vi "Client.vi"() -> ()   [LabVIEW 2025]
panel:
  in  "Stop":bool
  out "Waveform Chart":dbl(graph)
  out "Alarm Message":string
  out "Alarm LED":bool
  out "Max Temp":dbl
  out "Min Temp":dbl
  out "Moving Avg":dbl
  out "Current Temp":dbl
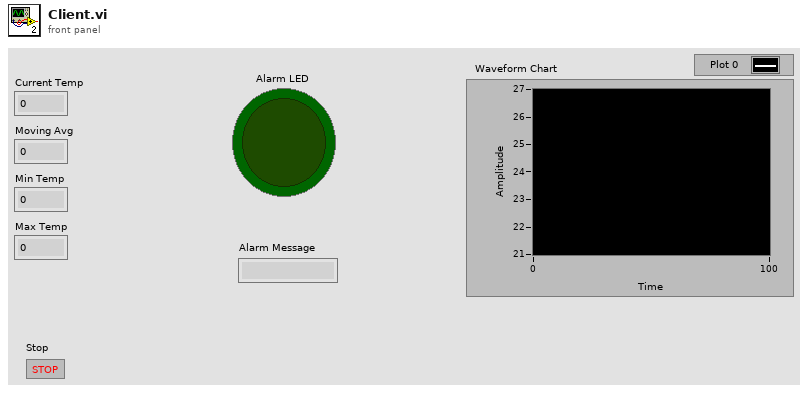
[diagram p1: front panel]
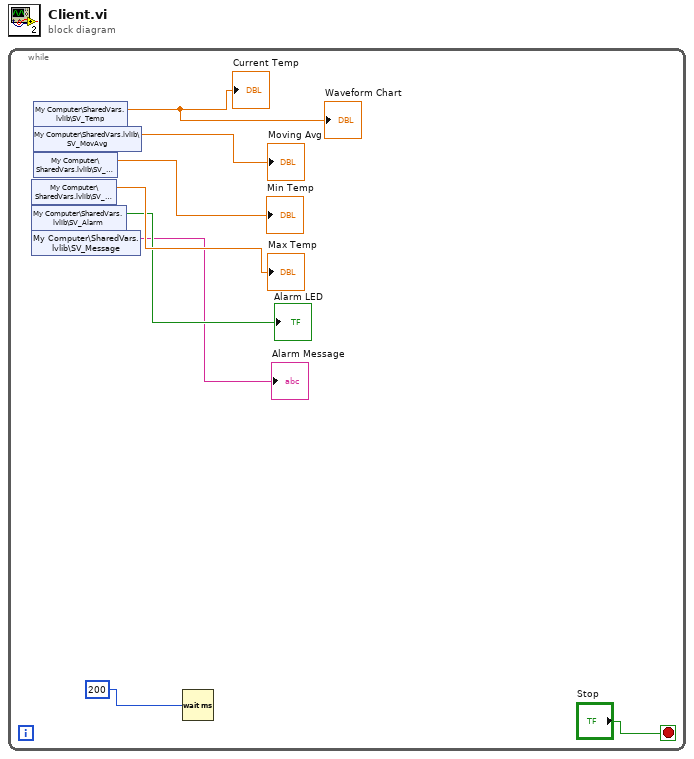
[diagram p0: block diagram]
diagram:
  n1 = while {
    stop <- "Stop" stop-if-true
    n2 = shared-variable "My Computer\\SharedVars.lvlib\\SV_Max"() -> (→"Max Temp":dbl)  [unwired: 1 in, 1 out]
    n3 = shared-variable "My Computer\\SharedVars.lvlib\\SV_Alarm"() -> (→"Alarm LED":bool)  [unwired: 1 in, 1 out]
    n4 = shared-variable "My Computer\\SharedVars.lvlib\\SV_Message"() -> (→"Alarm Message":string)  [unwired: 1 in, 1 out]
    n5 = shared-variable "My Computer\\SharedVars.lvlib\\SV_Temp"() -> (→"Current Temp" →"Waveform Chart":dbl)  [unwired: 1 in, 1 out]
    n6 = shared-variable "My Computer\\SharedVars.lvlib\\SV_MovAvg"() -> (→"Moving Avg":dbl)  [unwired: 1 in, 1 out]
    n7 = shared-variable "My Computer\\SharedVars.lvlib\\SV_Min"() -> (→"Min Temp":dbl)  [unwired: 1 in, 1 out]
    n8 = Wait (ms)(milliseconds to wait=200) -> ()  [unwired: 1 out]
  }
